vi "Read Loaded test recipe.vi"(8 "error in (no error)":errorcluster, 11 "Fiber Auto Collimation state data in":refnum<class "Fiber Auto Collimation state data.lvclass">) -> (0 "error out":errorcluster, 2 "Loaded test recipe":refnum<class "Test Recipe.lvclass">, 3 "Fiber Auto Collimation state data out":refnum<class "Fiber Auto Collimation state data.lvclass">)   [LabVIEW 2018, in "Fiber Auto Collimation state data.lvclass"]
doc: "Stores the currently loaded test recipe inside of the main station state data."
uses:
  Fiber Auto Collimation state data.lvclass
  <userlib>/Recipe/Test Recipe classes/Test Recipe.lvclass
  Fiber Auto Collimation state data.lvclass/Fiber Auto Collimation state data.ctl
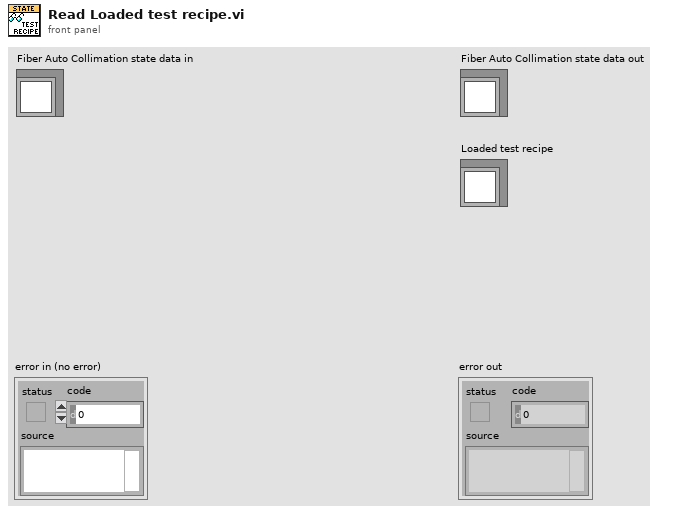
[diagram p1: front panel]
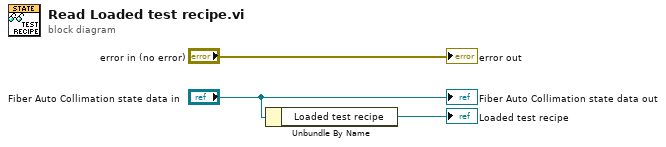
[diagram p0: block diagram]
diagram:
  n1 = Unbundle By Name("Fiber Auto Collimation state data in") -> ("Loaded test recipe"=→"Loaded test recipe":refnum<class "Test Recipe.lvclass">)
  "error out" <- "error in (no error)"
  "Fiber Auto Collimation state data out" <- "Fiber Auto Collimation state data in"
